vi "HAL camera get one frame.vi"(2 "error in":errorcluster, 3 "New Image":T1, 4 "Camera Parameters (important)":T2={"Exposure Time (sec)"=0.0, "EM CCD Gain"=0, "Readout Settings"={"Acquisition Mode"=enum."(do not use)", "Pixel Rate"=enum."EM CCD 30 Mhz 16 bits", "High Capacity?"=FALSE, "V Shift Speed (us/row)"=enum."0.6 (not reccommended)", "V Shift Amplitude"=enum."normal", "Preamp Gain"=enum."2", "Trigger Mode"=0, "Baseline offset"=0, "Baseline clamp"=FALSE}, "Image Size"={"H Bin"=0, "V Bin"=0, "Left"=0, "Top"=0, "Right"=0, "Bottom"=0}} {"Readout Settings"."Baseline offset" min=-1000 max=1000 step=100; "Readout Settings"."Trigger Mode" items=["Internal", "External"]; "EM CCD Gain" scale=1.0..300.0; "Exposure Time (sec)" scale=0.001..10.0 scale format="%#_1g"}) -> (0 "error out":errorcluster, 1 "Image Out":T1)   [LabVIEW 2016]
uses:
  ixon ultra 897/HAL camera parameters important.ctt
  ixon ultra 897/ixon readout settings.ctl
  ixon ultra 897/andor acquisition mode.ctl
  <vilib>/vision/Image Controls.llb/IMAQ Image.ctl
panel:
  # "Camera: Andor iXon Ultra"
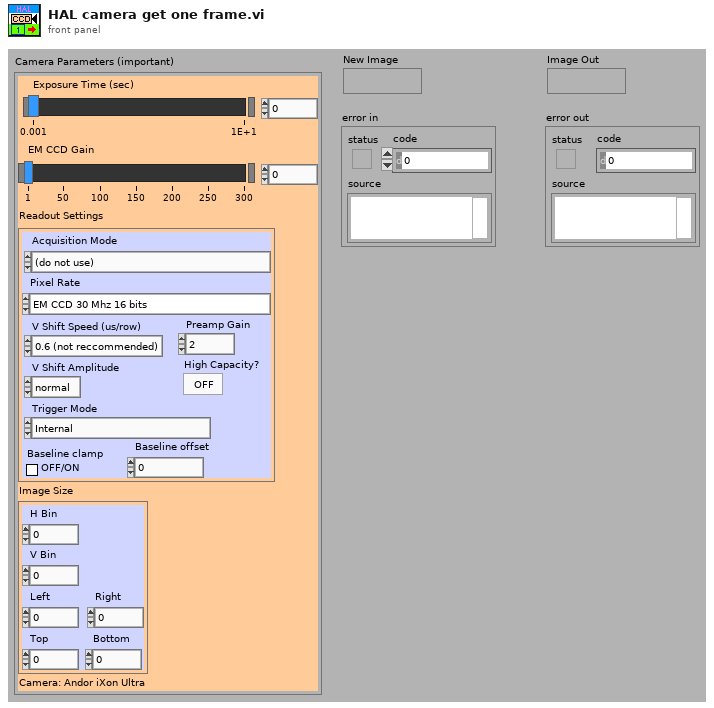
[diagram p1: front panel]
types:
  T1 = typedef "IMAQ Image.ctl" = refnum<image>
  T2 = typedef "HAL camera parameters important.ctt" = cluster{"Exposure Time (sec)":sgl, "EM CCD Gain":u16, "Readout Settings":T3, "Image Size":cluster{"H Bin":i32, "V Bin":i32, "Left":i32, "Top":i32, "Right":i32, "Bottom":i32}}
  T3 = typedef "ixon readout settings.ctl" = cluster{"Acquisition Mode":T4, "Pixel Rate":enum16{"EM CCD 30 Mhz 16 bits", "EM CCD 20 Mhz 16 bits", "EM CCD 10 Mhz 16 bits", "EM CCD 1 Mhz 16 bits", "Standard CCD 1 Mhz 16 bits", "Standard CCD 0.1 Mhz 16 bits"}, "High Capacity?":bool, "V Shift Speed (us/row)":enum16{"0.6 (not reccommended)", "1.13  (not reccommended)", "2.2  (not reccommended)", "4.33"}, "V Shift Amplitude":enum16{"normal", "+1", "+2", "+3", "+4"}, "Preamp Gain":enum16{"1", "2", "3"}, "Trigger Mode":u32, "Baseline offset":i16, "Baseline clamp":bool}
  T4 = typedef "andor acquisition mode.ctl" = enum16{"(do not use)", "Single Scan", "Accumulate", "Kinetics", "Fast Kinetics", "Kinetics Run till Abort", "Frame Transfer", "Frame Transfer Run till Abort", "(do not use) ", "Time Delayed Integration"}
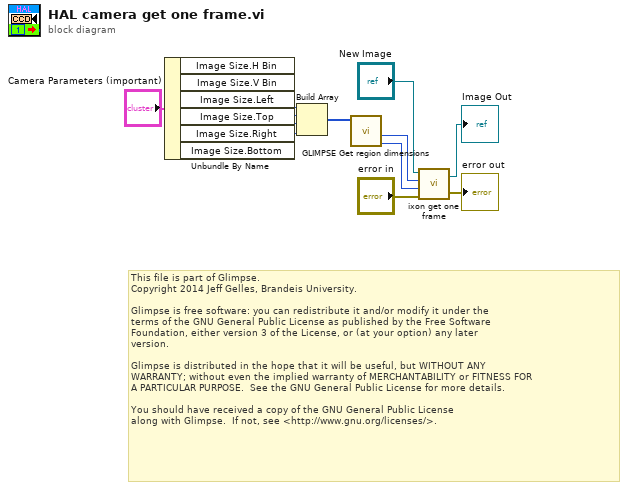
[diagram p0: block diagram]
diagram:
  # "This file is part of Glimpse. \nCopyright 2014 Jeff Gelles, Brandeis University.    \n\nGlimpse is free software: you can redistribute it and/or modify it under the \nterms of the GNU General Public License as published by the Free Software \nFoundation, either version 3 of the License, or (at your option) any later \nversion.\n\nGlimpse is distributed in the hope that it will be useful, but WITHOUT ANY \nWARRANTY; without even the implied warranty of MERCHANTABILITY or FITNESS FOR \nA PARTICULAR PURPOSE.  See the GNU General Public License for more details.\n\nYou should have received a copy of the GNU General Public License\nalong with Glimpse.  If not, see <http://www.gnu.org/licenses/>."
  n1 = Unbundle By Name("Camera Parameters (important)") -> ("Image Size.Left"=w10:i32, "Image Size.Top"=w9:i32, "Image Size.Right"=w8:i32, "Image Size.Bottom"=w7:i32)  [unwired: 2 out]
  n2 = Build Array(w10, w9, w8, w7) -> (w11:i32[])
  n3 = call "GLIMPSE Get region dimensions.vi"("x1y1x2y2"=w11) -> ("y size"=w2:u16, "x size"=w3:u16)  [unwired: 9 out]
  n4 = call "ixon get one frame.vi"("error in"="error in", "Image Height"=w2, "Image Width"=w3, "Image In"="New Image") -> ("error out"=→"error out":errorcluster, "Image Out"=→"Image Out":T1)  [unwired: 2 out]
